vi "AFM_Driver_Manager.SendLithography.vi"(8 "error in (no error)":errorcluster, 10 "Lithography Data":T2(array[cluster]), 11 "AFM_Driver_Manager in":refnum<class "AFM_Driver_Manager.lvclass">) -> (0 "error out":errorcluster, 3 "AFM_Driver_Manager out":refnum<class "AFM_Driver_Manager.lvclass">)   [LabVIEW 2019, in "AFM_Driver_Manager.lvclass"]
uses:
  AFM_Driver_Manager.lvclass
  <userlib>/LevyLab/Relay Box/Typedefs/Resistor--enum.ctl
  <userlib>/LevyLab/Relay Box/Relay-Box.lvclass
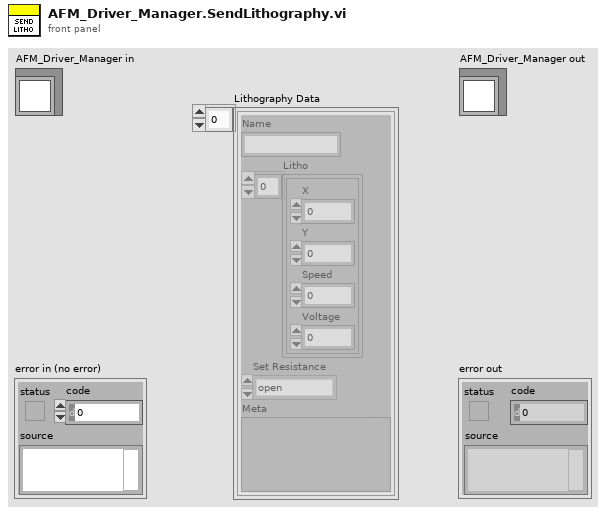
[diagram p1: front panel]
types:
  T1 = typedef "Relay-Box.lvclass/Resistor--enum.ctl" = enum16{"open", "discharge tip", "0 ohms", "100k ohm", "10M ohm", "1G ohm"}
  T2 = cluster{"Name":string, "Litho":cluster{"X":dbl, "Y":dbl, "Speed":dbl, "Voltage":dbl}[], "Set Resistance":T1, "Meta":variant}[]
  T3 = typedef "AFM_Driver_Manager.lvclass/AFM_Driver_Manager.PublicMethods.ctl" = cluster{"Stop Event":refnum<user-event>, "Lithography Data":refnum<user-event>, "Run Lithography":refnum<user-event>, "Background Image":refnum<user-event>, "Abort Notifier":refnum<user-event>}
  T4 = cluster{"VI Refnum":refnum<vi>, "Path":path, "Name":string, "Events":T3}
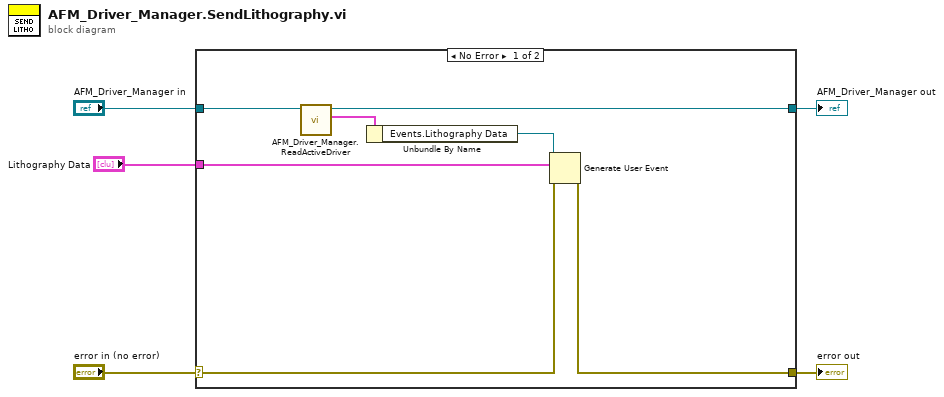
[diagram p0: block diagram]
diagram:
  n1 = case shown="No Error" "error in (no error)" {
    selector: "error in (no error)" -> [w8 w14]
    tunnel: [w7 w14] -> w4
    tunnel: [w12 w13] -> w2
    tunnel: "AFM_Driver_Manager in" -> [w11 w13]
    tunnel: "Lithography Data" -> [w9 _]
    frame No Error {
      n2 = call "AFM_Driver_Manager.ReadActiveDriver.vi"("AFM_Driver_Manager in"=w11) -> ("Active Driver"=w10:T4, "AFM_Driver_Manager out"=w12:refnum<class "AFM_Driver_Manager.lvclass">)  [unwired: 8 in, 1 out]
      n3 = Unbundle By Name(w10) -> ("Events.Lithography Data"=w6:refnum<user-event>)
      n4 = Generate User Event(user event=w6, event data cluster=w9, error in=w8) -> (error out=w7:errorcluster)  [unwired: 1 in, 1 out]
    }
    frame Error {
    }
  }
  "error out" <- w4
  "AFM_Driver_Manager out" <- w2
